vi "Read register.vi"(8 "error in (no error)":errorcluster, 11 "PLCMonitor in":refnum<class "PLCMonitor.lvclass">) -> (0 "error out":errorcluster, 3 "PLCMonitor out":refnum<class "PLCMonitor.lvclass">)   [LabVIEW 2020, in "PLCMonitor.lvlib" / "PLCMonitor.lvclass"]
uses:
  PLCMonitor.lvclass
  C:/Program Files/National Instruments/LabVIEW 2020/vi.lib/gpm_packages/@cs/mva-core/Source/IModel/IModel/IModel.lvclass
  PLCMonitor.lvclass/PLCMonitor.ctl
  <vilib>/gpm_packages/@cs/mva-core/Source/IObserver/IObserver/IObserver.lvclass/IObserver.ctl
  <vilib>/gpm_packages/@cs/mva-core/Source/IModel/IModel/IModel.lvclass/IModel.ctl
  <vilib>/gpm_packages/@cs/mva-core/Source/IMediator/PublishRequest/PublishRequest.lvclass/PublishRequest.ctl
  <vilib>/gpm_packages/@cs/mva-core/Source/IMediator/IMediator Messages/Publish Msg/Publish Msg.lvclass/Publish Msg.ctl
  <vilib>/gpm_packages/@cs/actor-framework-messages/Source/RoundTripMessage/RoundTripMessage.lvclass/RoundTripMessage.ctl
  <vilib>/ActorFramework/Message Enqueuer/Message Enqueuer.lvclass/Message Enqueuer.ctl
  <vilib>/gpm_packages/@cs/mva-core/Source/IMediator/IMediator Messages/Publish Msg/Send Pre-Addressed Publish.vi
  <vilib>/gpm_packages/@cs/mva-core/Source/IObserver/IObserver/Read Unique ID.vi
  <vilib>/gpm_packages/@cs/mva-core/Source/IMediator/PublishRequest/Pack Publish Request.vi
  <vilib>/gpm_packages/@cs/actor-framework-messages/Source/RoundTripMessage/Return Round-Trip Message.vi
  <vilib>/ActorFramework/Message Enqueuer/Enqueue.vi
  <vilib>/gpm_packages/@cs/mva-core/Source/IModel/IModel/IModel.lvclass
  C:/Program Files/National Instruments/LabVIEW 2020/vi.lib/gpm_packages/@cs/mva-core/Source/IObserver/IObserver/IObserver.lvclass
  <vilib>/gpm_packages/@cs/mva-core/Source/IMediator/IMediator Messages/Publish Msg/Publish Msg.lvclass
  C:/Program Files/National Instruments/LabVIEW 2020/vi.lib/gpm_packages/@cs/actor-framework-messages/Source/RoundTripMessage/RoundTripMessage.lvclass
  <vilib>/gpm_packages/@cs/actor-framework-messages/Source/RoundTripMessage/RoundTripMessage.lvclass
  C:/Program Files/National Instruments/LabVIEW 2020/vi.lib/ActorFramework/Message/Message.lvclass
  <vilib>/Utility/error.llb/Error Cluster From Error Code.vi
  <vilib>/ActorFramework/Message Priority Queue/Priority Enqueue.vi
  <vilib>/gpm_packages/@cs/mva-core/Source/IMediator/PublishRequest/PublishRequest.lvclass
  HslCommunication/Abstract PLC Controler/Abs Controler.lvclass
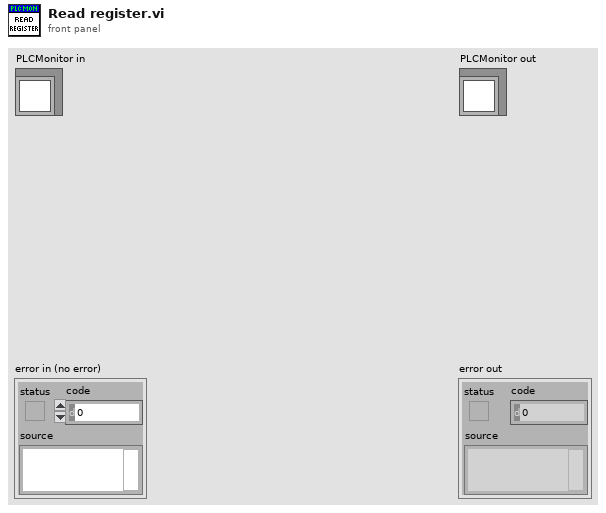
[diagram p1: front panel]
types:
  T1 = typedef "PLCMonitor.lvlib/Read Config.ctl" = cluster{"Start address":string, "length":u16, "Data type":T2}
  T2 = typedef "PLCMonitor.lvlib/DataType.ctl" = enum8{"Invalid Type", "Void", "I16", "I32", "I64", "U16", "U32", "U64", "Single Float", "Double Float", "Boolean", "String"}
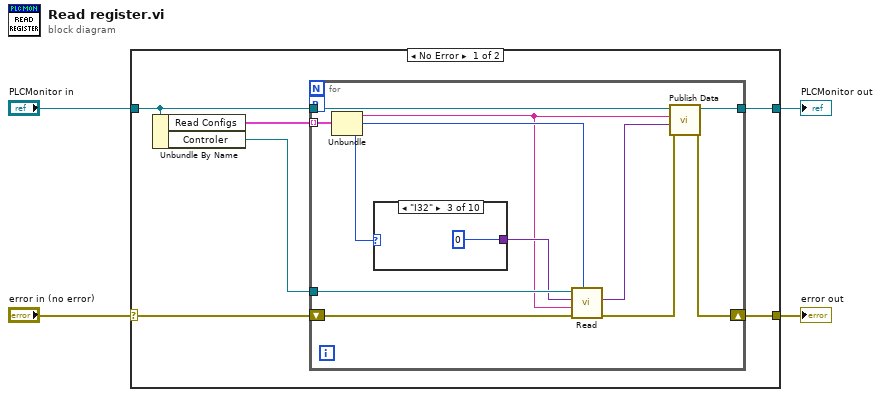
[diagram p0: block diagram]
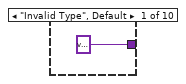
[diagram p2: hidden frame]
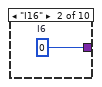
[diagram p3: hidden frame]
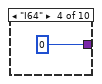
[diagram p4: hidden frame]
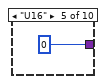
[diagram p5: hidden frame]
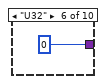
[diagram p6: hidden frame]
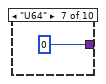
[diagram p7: hidden frame]
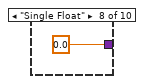
[diagram p8: hidden frame]
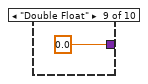
[diagram p9: hidden frame]
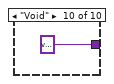
[diagram p10: hidden frame]
diagram:
  n1 = case shown="No Error" "error in (no error)" {
    selector: "error in (no error)" -> [w10 w34]
    tunnel: [w9 w34] -> w3
    tunnel: [w6 w33] -> w1
    tunnel: "PLCMonitor in" -> [w5 w33]
    frame No Error {
      n2 = Unbundle By Name(w5) -> ("Read Configs"=w7:T1[], "Controler"=w8:refnum<class "Abs Controler.lvclass">)
      n3 = for {
        tunnel: w8 -> [w21]
        shift-right: [w11] -> w9
        shift-left: w10 -> [w22]
        tunnel: w7 -> [w20] mode=indexing
        tunnel: w5 -> [w16]
        tunnel: [w15] -> w6
        workers-P: _ -> [_]
        n4 = Unbundle(w20) -> ("Start address"=w14:string, "length"=w19:u16, "Data type"=w18:T2)
        n5 = case shown="\"I32\"" w18 {
          tunnel: [variant w24 0 ("I6") i64 0 ("I6") u16 0 ("I6") u32 0 ("I6") u64 0 ("I6") sgl 0.0 ("I6") 0.0 ("I6") variant ("I6")] -> w17
          frame "Invalid Type", Default {
          }
          frame "I16" {
            w24 = i16 0  # I6
          }
          frame "I32" {
          }
          frame "I64" {
          }
          frame "U16" {
          }
          frame "U32" {
          }
          frame "U64" {
          }
          frame "Single Float" {
          }
          frame "Double Float" {
          }
          frame "Void" {
          }
        }
        n6 = call-dynamic "Read.vi"("length"=w19, "error in (no error)"=w22, "Start address"=w14, "Read Type"=w17, "MelsecTCP in"=w21) -> ("error out"=w12:errorcluster, "Data"=w13:variant)  [unwired: 4 in, 1 out]
        n7 = call <vilib>:"Publish Data.vi"("error in (no error)"=w12, "Data to Publish"=w13, "Datum Name"=w14, "IModel in"=w16) -> ("error out"=w11:errorcluster, "IModel out"=w15:refnum<class "PLCMonitor.lvclass">)  [unwired: 6 in]
      }
    }
    frame Error {
    }
  }
  "error out" <- w3
  "PLCMonitor out" <- w1
